vi "Send.vi"(7 "path override":path, 8 "error in (no error)":errorcluster, 9 "flags_":i32, 10 "buf":string, 11 "s":u64) -> (0 "error out":errorcluster, 3 "s_":u64)   [LabVIEW 2025, in "libzmq-v143-mt-4_3_6.lvlib"]
uses:
  libzmq-v143-mt-4_3_6.lvlib
  errno.vi
  strerror.vi
  <vilib>/Utility/error.llb/Error Cluster From Error Code.vi
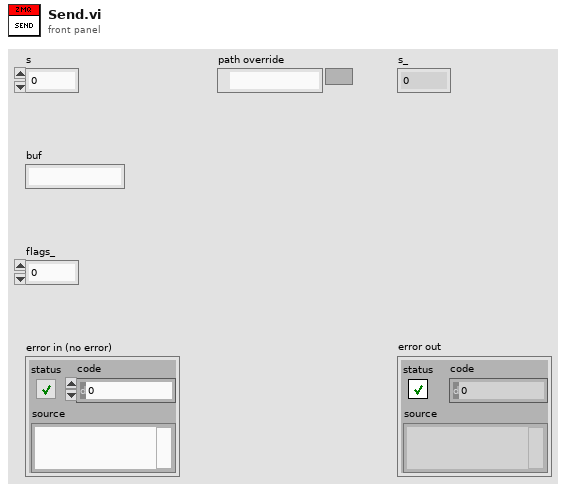
[diagram p1: front panel]
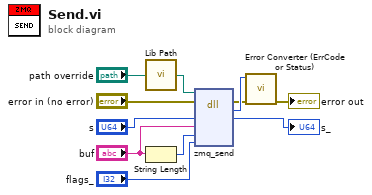
[diagram p0: block diagram]
diagram:
  n1 = call "Lib Path.vi"("path override"="path override") -> ("lib path"=w1:path)
  n2 = String Length(string="buf") -> (length=w4:i32)
  n3 = dll-call lib="home/james/Documents/ZeroMQ_LV/libzmq-v143-mt-4_3_6/libzmq.so" fn="zmq_send"(path in=w1, error in="error in (no error)", "s_"="s", "buf"="buf", "len"=w4, "flags_"="flags_") -> (error out=w10:errorcluster, "return type"=w11:i32, "s_"=→"s_":u64)  [unwired: 4 in, 1 out]
  n4 = call "Error Converter (ErrCode or Status).vi"("error in (no error)"=w10, "error code"=w11) -> ("error out"=→"error out":errorcluster)  [unwired: 9 in]
